vi "PreTipShapingCheck.vi"(11 "Input":string="34,45,89") -> (1 "error":bool, 2 "Error":errorcluster, 3 "concatenated error":string)   [LabVIEW 2014]
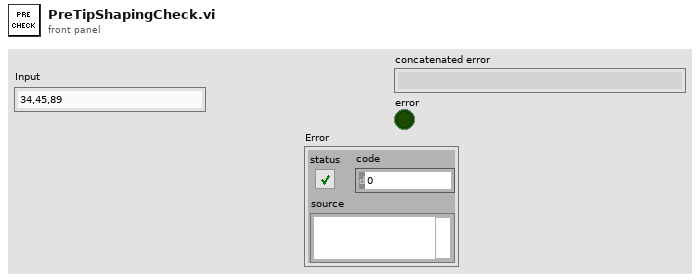
[diagram p1: front panel]
types:
  T1 = enum16{"pixel", "position", "size", "dip", "bias", "timing"}
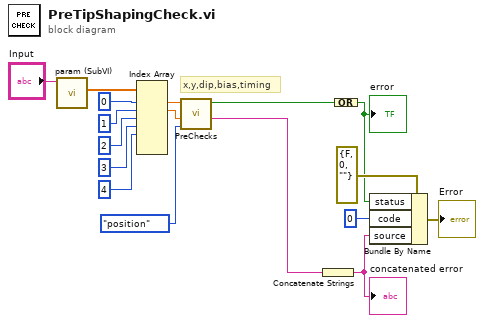
[diagram p0: block diagram]
diagram:
  # "x,y,dip,bias,timing"
  n1 = call <userlib>:"param (SubVI).vi"("Input"="Input") -> ("parm"=w17:dbl[])  [unwired: 8 in, 2 out]
  n2 = Index Array(array=w17, index #1=0 ("index"), index #2=1 ("index"), index #3=2 ("index"), index #4=3 ("index"), index #5=4 ("index")) -> (element #1=w11:dbl, element #2=w10:dbl)  [unwired: 2 in, 5 out]
  n3 = call "PreChecks.vi"("type"=T1."position", "Y"=w10, "X"=w11) -> ("message"=w9:string, "Error"=w8:bool)  [unwired: 7 in]
  n4 = Concatenate Strings(w9) -> (w5:string)
  "concatenated error" <- w5
  n5 = Compound Arithmetic op=OR(w8) -> (w6:bool)
  "error" <- w6
  n6 = Bundle By Name(cluster=errorcluster {"status"=FALSE, "code"=0, "source"=""} ("error in (no error)"), "status"=w6, "code"=0, "source"=w5) -> (→"Error":errorcluster)
